vi "Controle_vacuo.vi"(3 "time (s) to wait vacuo":u32=30000, 11 "Boolean":bool=TRUE) -> (8 "Vacuo":bool)   [LabVIEW 2011]
uses:
  <vilib>/Utility/error.llb/DialogType.ctl
  <vilib>/DAQmx/write.llb/DAQmx Write (Digital Bool 1Line 1Point).vi
  <vilib>/DAQmx/create/channels.llb/DAQmx Create Channel (DO-Digital Output).vi
  <vilib>/DAQmx/miscellaneous.llb/DAQmx Fill In Error Info.vi
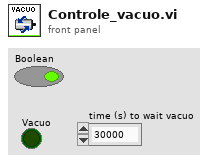
[diagram p1: front panel]
types:
  T1 = typedef "DialogType.ctl" = u16
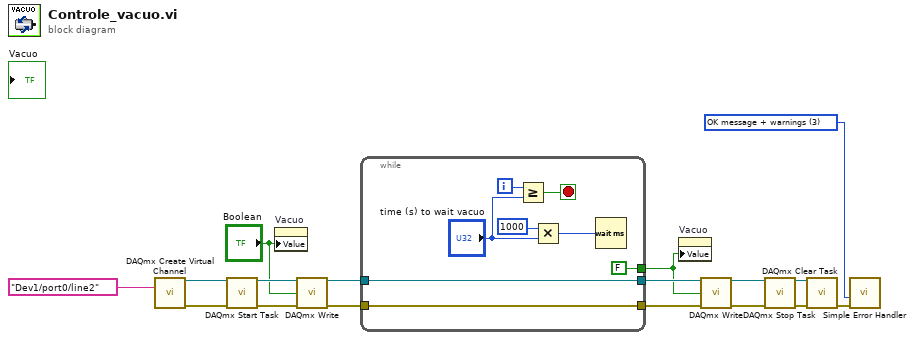
[diagram p0: block diagram]
diagram:
  w14 = T1 3 items=["no dialog", "OK message", "continue or stop message", "OK message + warnings", "continue/stop + warnings"] ("type of dialog (OK msg:1)")
  n1 = call-poly <vilib>:"DAQmx Create Virtual Channel.vi"("lines"=tag "Dev1/port0/line2") -> ("task out"=w16:refnum<k21>, "error out"=w15:errorcluster)  [unwired: 13 in]
  n2 = call <vilib>:"DAQmx Start Task.vi"("task/channels in"=w16, "error in"=w15) -> ("task out"=w13:refnum<k21>, "error out"=w12:errorcluster)  [unwired: 12 in]
  n3 = property on="Vacuo" class="Bool (strict)"("Value"="Boolean") -> ()  [unwired: 2 in, 2 out]
  n4 = call-poly <vilib>:"DAQmx Write.vi"("task/channels in"=w13, "data"="Boolean", "error in"=w12) -> ("task out"=w7:refnum<k21>, "error out"=w4:errorcluster)  [unwired: 10 in, 1 out]
  n5 = while {
    tunnel: [FALSE ("Boolean")] -> w2
    tunnel: [w22] -> w6
    tunnel: w7 -> [w22]
    tunnel: [w21] -> w5
    tunnel: w4 -> [w21]
    i -> [w20]
    stop <- w18 stop-if-true
    n6 = Greater Or Equal?(x=w20, y="time (s) to wait vacuo") -> (x >= y?=w18:bool)
    n7 = Multiply(x=u32 1000, y="time (s) to wait vacuo") -> (x*y=w24:u32)
    n8 = Wait (ms)(milliseconds to wait=w24) -> ()  [unwired: 1 out]
  }
  n9 = property on="Vacuo" class="Bool (strict)"("Value"=w2) -> ()  [unwired: 2 in, 2 out]
  n10 = call-poly <vilib>:"DAQmx Write.vi"("task/channels in"=w6, "data"=w2, "error in"=w5) -> ("task out"=w9:refnum<k21>, "error out"=w8:errorcluster)  [unwired: 10 in, 1 out]
  n11 = call <vilib>:"DAQmx Stop Task.vi"("task/channels in"=w9, "error in"=w8) -> ("task out"=w10:refnum<k21>, "error out"=w11:errorcluster)  [unwired: 12 in]
  n12 = call <vilib>:"DAQmx Clear Task.vi"("task in"=w10, "error in"=w11) -> ("error out"=w17:errorcluster)  [unwired: 13 in]
  n13 = call <vilib>:"Simple Error Handler.vi"("type of dialog (OK msg:1)"=w14, "error in (no error)"=w17) -> ()  [unwired: 3 in, 5 out]
